vi "UserSliderCursor (SubVI).vi"(6 "Axes colour":u32(colorbox)=16711680, 8 "error in (no error)":errorcluster, 9 "Image RefNum In":T1, 10 "Y slider refnum":refnum<vi>, 11 "X slider refnum":refnum<vi>) -> (0 "error out":errorcluster, 2 "Image Refnum out":T1, 3 "Cross Point":cluster{"X coordinate":dbl, "Y coordinate":dbl})   [LabVIEW 2016]
uses:
  <vilib>/vision/Image Controls.llb/IMAQ Image.ctl
  <resource>/objmgr/IMAQImage.rc
panel:
  # "This subVI takes input from a pair of \nsliders to display axes on an image. \nThe Cross Point provides the \n(x,y) coordinates of the intersection\nof the two axes (in pixel units)"
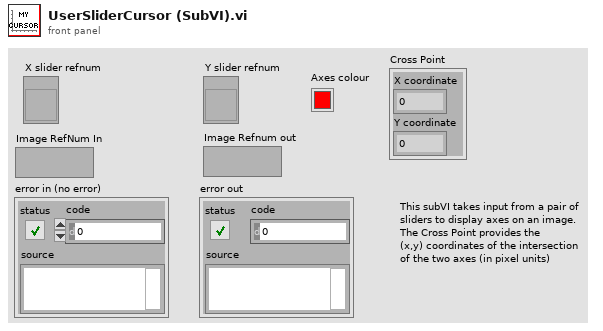
[diagram p1: front panel]
types:
  T1 = typedef "IMAQ Image.ctl" = refnum<image>
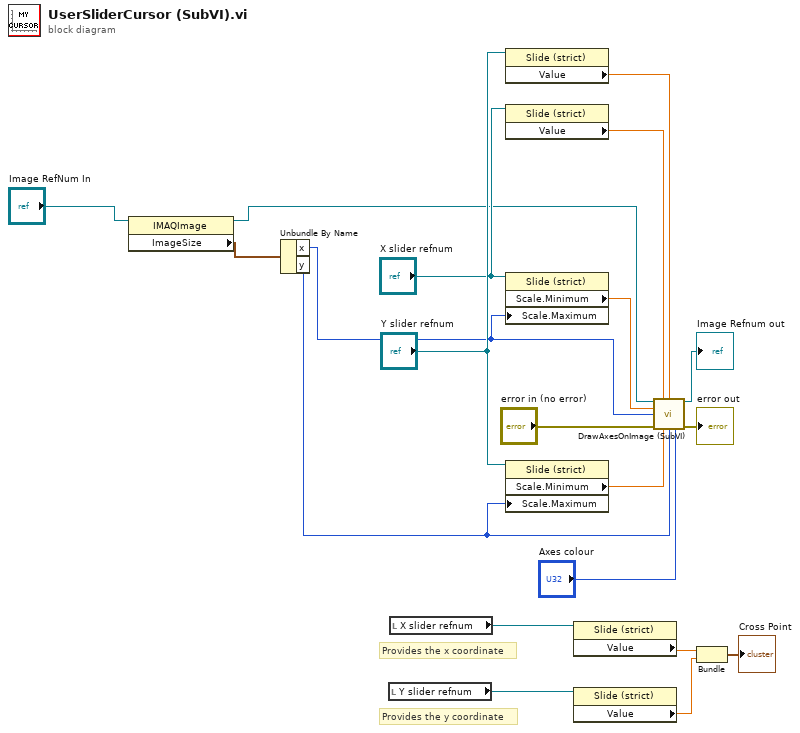
[diagram p0: block diagram]
diagram:
  # "Provides the x coordinate"
  # "Provides the y coordinate"
  n1 = property class="IMAQImage"(reference="Image RefNum In") -> (reference out=w3:T1, "ImageSize"=w5:cluster{"x":i32, "y":i32})  [unwired: 1 in, 1 out]
  n2 = Unbundle By Name(w5) -> ("x"=w2:i32, "y"=w1:i32)
  n3 = local read "Y slider refnum"() -> (w9:refnum<vi>)
  n4 = local read "X slider refnum"() -> (w10:refnum<vi>)
  n5 = property class="Slide (strict)"(reference="Y slider refnum") -> ("Value"=w12:dbl)  [unwired: 1 in, 2 out]
  n6 = property class="Slide (strict)"(reference="X slider refnum") -> ("Value"=w11:dbl)  [unwired: 1 in, 2 out]
  n7 = property on="Property Node" class="Slide (strict)"(reference="X slider refnum", "Scale.Maximum"=w2) -> ("Scale.Minimum"=w13:dbl)  [unwired: 1 in, 2 out]
  n8 = property on="Property Node" class="Slide (strict)"(reference="Y slider refnum", "Scale.Maximum"=w1) -> ("Scale.Minimum"=w14:dbl)  [unwired: 1 in, 2 out]
  n9 = property class="Slide (strict)"(reference=w10) -> ("Value"=w7:dbl)  [unwired: 1 in, 2 out]
  n10 = property class="Slide (strict)"(reference=w9) -> ("Value"=w6:dbl)  [unwired: 1 in, 2 out]
  n11 = call "DrawAxesOnImage (SubVI).vi"("Image Refnum in"=w3, "X Value"=w11, "Y Value"=w12, "X Minimum"=w13, "X Maximum"=w2, "error in (no error)"="error in (no error)", "Y Minimum"=w14, "Y Maximum"=w1, "Axes colour"="Axes colour") -> ("Image Refnum out"=→"Image Refnum out":T1, "error out"=→"error out":errorcluster)  [unwired: 5 in]
  n12 = Bundle("Value"=w7, "Value"=w6) -> (→"Cross Point":cluster{"Value":dbl, "Value":dbl})  [unwired: 1 in]
